vi "matrici_v40.vi"() -> ()   [LabVIEW 2009]
uses:
  <vilib>/Math Plots/3D Math Plots/3D Surface/3D Surface XCtrl/3D Surface.xctl
  <vilib>/Math Plots/3D Math Plots/3D Surface/3D Surface Datatype/3D Surface Datatype.lvclass
  <vilib>/Math Plots/3D Math Plots/3D Surface/3D Surface Datatype/Public/Plot Helper (Vector).vi
panel:
  out "y":dbl=1.9999999999999982
  out "X":dbl=1.9999999999999982
  out "3D Surface":refnum<class "3D Plot Datatype.lvclass">[](xcontrol)
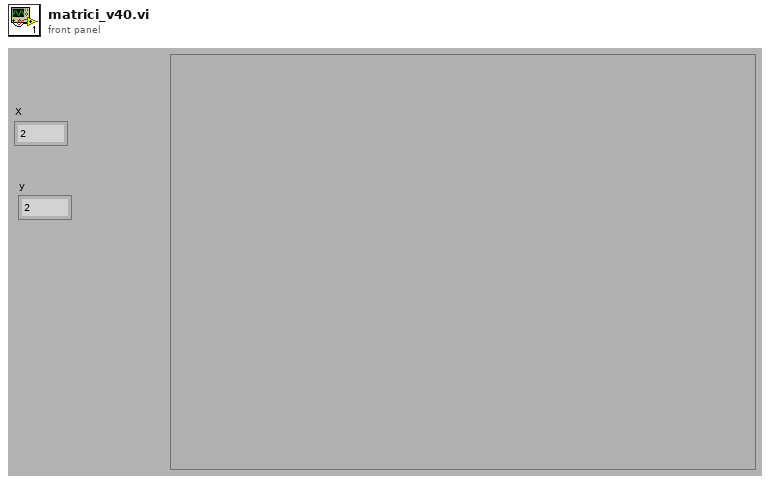
[diagram p1: front panel]
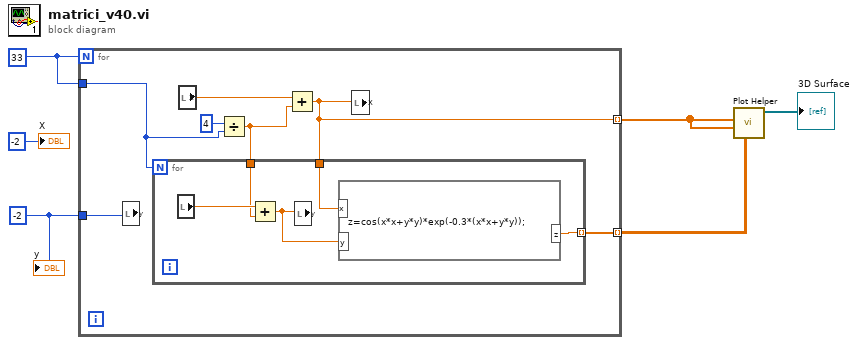
[diagram p0: block diagram]
diagram:
  w5 = 33
  w4 = -2
  n1 = for {
    N: w5 -> [_]
    tunnel: [w12] -> w2 mode=indexing
    tunnel: [w11] -> w1 mode=indexing
    tunnel: w5 -> [w9]
    tunnel: w4 -> [w7]
    n2 = local write "y"(w7) -> ()
    n3 = local read "X"() -> (w13:dbl)
    n4 = Divide(x=4, y=w9) -> (x/y=w8:dbl)
    n5 = Add(x=w13, y=w8) -> (x+y=w12:dbl)
    n6 = for {
      N: w9 -> [_]
      tunnel: w12 -> [w17]
      tunnel: [w15] -> w11 mode=indexing
      tunnel: w8 -> [w14]
      n7 = local read "y"() -> (w18:dbl)
      n8 = Add(x=w18, y=w14) -> (x+y=w16:dbl)
      n9 = local write "y"(w16) -> ()
      n10 = formula code="z=cos(x*x+y*y)*exp(-0.3*(x*x+y*y));"("x"=w17, "y"=w16) -> ("z"=w15:dbl)
    }
    n11 = local write "X"(w12) -> ()
  }
  n12 = call-poly <vilib>:"Plot Helper.vi"("z matrix"=w1, "y vector"=w2, "x vector"=w2) -> ("3D Plot lvclass Array out"=→"3D Surface":refnum<class "3D Plot Datatype.lvclass">[])  [unwired: 3 in, 5 out]
  "X" <- -2
  "y" <- w4
